vi "DCA Build Key Array for Config.vi"(8 "error in (no error)":errorcluster, 9 "DC Attenuation Test Parameters":T2={"Stimulus"={"Use Instrument"=FALSE, "Normalize"=FALSE, "Blank Screen"=FALSE, "Measurement Type"=enum."Diode", "Range"=enum."Auto", "Resolution"=enum."Auto"}, "Measurement"={"Topology"=enum."PI-Network", "Lock Topology"=FALSE, "ATTN Calc"=enum."Power", "Zo"=50.0}, "Limits"=[], "Normalization"={"Normalized?"=FALSE, "Rab Value"=0.0, "Rac Value"=0.0, "Rbc Value"=0.0}}, 10 "Key Array In":T13, 11 "Connection Refnum":T1) -> (0 "error out":errorcluster, 1 "$$INITCODE$$":string, 2 "Key Array Out":T13, 3 "Connection Refnum":T1)   [LabVIEW 2011]
uses:
  ITK EXT/utils/keyedarr.llb/Keyed Array.ctl
  TypeDefs/DCA Test Parameters.ctl
  TypeDefs/DCA Stimulus Parameters.ctl
  TypeDefs/DCA Measurement Cluster.ctl
  TypeDefs/DCA Topology.ctl
  TypeDefs/DCA Attenuation Calculation.ctl
  TypeDefs/DCA Limit.ctl
  TypeDefs/DCA Limit Quantity.ctl
  TypeDefs/DCA Limit Comparison.ctl
  TypeDefs/DCA Limit Operation.ctl
  Test Referential Limit.ctl
  TypeDefs/DCA Calibration State.ctl
  Summitek EXT/ODBC/SQL Controls/Connection Refnum.ctl
  ITK EXT/utils/strutil.llb/Case Matching.ctl
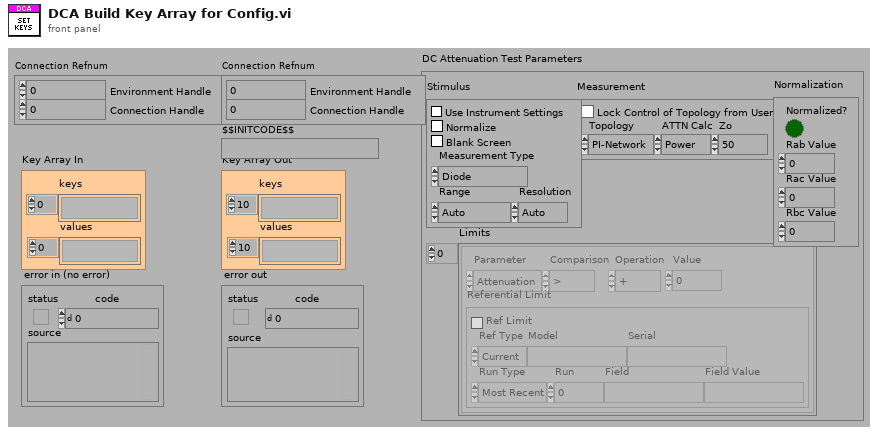
[diagram p1: front panel]
types:
  T1 = typedef "Connection Refnum.ctl" = cluster{"Environment Handle":i32, "Connection Handle":i32}
  T2 = typedef "DCA Test Parameters.ctl" = cluster{"Stimulus":T3, "Measurement":T4, "Limits":T7[], "Normalization":T12}
  T3 = typedef "DCA Stimulus Parameters.ctl" = cluster{"Use Instrument":bool, "Normalize":bool, "Blank Screen":bool, "Measurement Type":enum16{"Voltage DC", "Voltage DC Ratio", "Voltage AC", "Current DC", "Current AC", "Resistance", "Fresistance", "Frequency", "Period", "Continuity", "Diode"}, "Range":enum16{"Auto", "Minimum", "Maximum", "100", "1,000", "10,000", "100,000", "1,000,000", "10,000,000", "100,000,000"}, "Resolution":enum16{"Auto", "4 1/2", "5 1/2", "6 1/2"}}
  T4 = typedef "DCA Measurement Cluster.ctl" = cluster{"Topology":T5, "Lock Topology":bool, "ATTN Calc":T6, "Zo":dbl}
  T5 = typedef "DCA Topology.ctl" = enum32{"PI-Network", "T-Network"}
  T6 = typedef "DCA Attenuation Calculation.ctl" = enum32{"Power", "Voltage"}
  T7 = typedef "DCA Limit.ctl" = cluster{"Parameter":T8, "Comparison":T9, "Operation":T10, "Value":dbl, "Referential Limit":T11}
  T8 = typedef "DCA Limit Quantity.ctl" = enum16{"Attenuation", "Zin", "Zout", "R1", "R2", "R3", "Rab", "Rac", "Rbc"}
  T9 = typedef "DCA Limit Comparison.ctl" = enum16{">", ">=", "<", "<="}
  T10 = typedef "DCA Limit Operation.ctl" = enum16{"+", "-"}
  T11 = typedef "Test Referential Limit.ctl" = cluster{"Ref Limit":bool, "Ref Type":enum16{"Current", "Specify"}, "Model":string, "Serial":string, "Run Type":enum16{"Most Recent", "Run #", "Match Field"}, "Run":i32, "Field":string, "Field Value":string}
  T12 = typedef "DCA Calibration State.ctl" = cluster{"Normalized?":bool, "Rab Value":dbl, "Rac Value":dbl, "Rbc Value":dbl}
  T13 = typedef "Keyed Array.ctl" = cluster{"keys":string[], "values":string[]}
  T14 = typedef "Case Matching.ctl" = enum16{"a != A", "a == A", "system"}
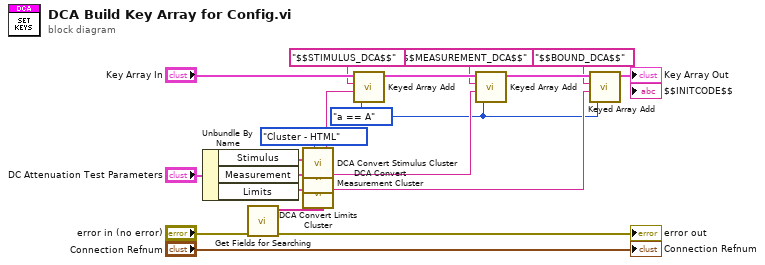
[diagram p0: block diagram]
diagram:
  w8 = enum16{"Cluster - HTML", "HTML - Cluster"}."Cluster - HTML" ("Conversion")
  w4 = Case_Matching."a == A" ("case matching (sensitive)")
  n1 = Unbundle By Name("DC Attenuation Test Parameters") -> ("Stimulus"=w9:T3, "Measurement"=w16:T4, "Limits"=w10:T7[])
  n2 = call "Get Fields for Searching.vi"("error in"="error in (no error)") -> ("error out"=→"error out":errorcluster, "Field Records List"=w11:string[])  [unwired: 9 out]
  n3 = call "DCA Convert Stimulus Cluster.vi"("Conversion"=w8, "Stimulus Cluster In"=w9) -> ("Stumulus HTML Out"=w2:string)  [unwired: 1 in, 5 out]
  n4 = call "DCA Convert Measurement Cluster.vi"("Conversion"=w8, "Measurements Cluster In"=w16) -> ("Measurements HTML Out"=w17:string)  [unwired: 1 in, 5 out]
  n5 = call "DCA Convert Limits Cluster.vi"("Fields Names"=w11, "Conversion"=w8, "Limits Cluster In"=w10) -> ("Limits HTML Out"=w15:string)  [unwired: 1 in, 5 out]
  n6 = call "Keyed Array Add.vi"("case matching (sensitive)"=w4, "value"=w2, "key"="$$STIMULUS_DCA$$", "array in"="Key Array In") -> ("array out"=w5:T13)  [unwired: 3 out]
  n7 = call "Keyed Array Add.vi"("case matching (sensitive)"=w4, "value"=w17, "key"="$$MEASUREMENT_DCA$$", "array in"=w5) -> ("array out"=w19:T13)  [unwired: 3 out]
  n8 = call "Keyed Array Add.vi"("case matching (sensitive)"=w4, "value"=w15, "key"="$$BOUND_DCA$$", "array in"=w19) -> ("array out"=→"Key Array Out":T13)  [unwired: 3 out]
  "Connection Refnum" <- "Connection Refnum"
